vi "Combo box Read Write Strings.vi"(8 "error in (no error)":errorcluster, 9 "Enum":enum16{"Read", "Write"}(ring)=enum."Write", 10 "Strings []":string[](array[string]), 11 "ComboBox in":refnum<vi>) -> (0 "error out":errorcluster, 3 "Strings[]Out":string[](array[string]))   [LabVIEW 2018]
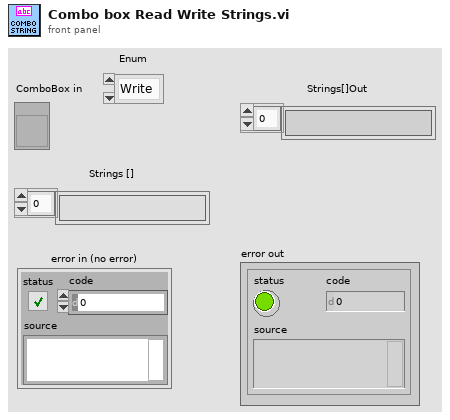
[diagram p1: front panel]
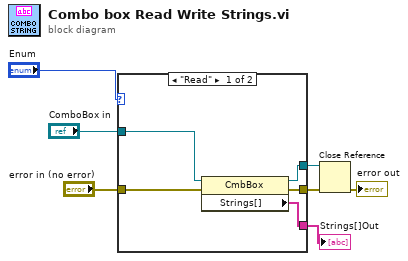
[diagram p0: block diagram]
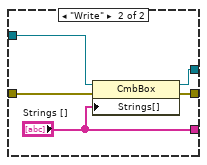
[diagram p2: hidden frame]
diagram:
  n1 = case shown="\"Read\"" "Enum" {
    tunnel: "ComboBox in" -> [w12 w17]
    tunnel: [w10 w16] -> w2
    tunnel: [w9 w15] -> w3
    tunnel: "error in (no error)" -> [w11 w14]
    tunnel: [w8 "Strings []"] -> w7
    frame "Read" {
      n2 = property class="CmbBox"(reference=w12, error in=w11) -> (reference out=w10:refnum<vi>, error out=w9:errorcluster, "Strings[]"=w8:string[])
    }
    frame "Write" {
      n3 = property class="CmbBox"(reference=w17, error in=w14, "Strings[]"="Strings []") -> (reference out=w16:refnum<vi>, error out=w15:errorcluster)
    }
  }
  "Strings[]Out" <- w7
  n4 = Close Reference(reference=w2, error in (no error)=w3) -> (error out=→"error out":errorcluster)
